vi "SensorInit.vi"(8 "error in (no error)":errorcluster, 9 "TC channel":tag="cDAQ1Mod3/ai0,cDAQ1Mod3/ai1,cDAQ1Mod3/ai2,cDAQ1Mod3/ai3,cDAQ1Mod3/ai4,cDAQ1Mod3/ai5,cDAQ1Mod3/ai6,cDAQ1Mod3/ai7", 10 "physical channels in":tag="cDAQ1Mod1/ai1,cDAQ1Mod1/ai2", 11 "Sample Rate":dbl) -> (0 "error out":errorcluster, 3 "Task out":refnum<k21>)   [LabVIEW 2020]
uses:
  <vilib>/DAQmx/create/channels.llb/DAQmx Create Channel (AI-Temperature-Thermocouple).vi
  <vilib>/DAQmx/create/channels.llb/DAQmx Create Channel (AI-Voltage-Basic).vi
  <vilib>/DAQmx/configure/timing.llb/DAQmx Timing (Sample Clock).vi
  <resource>/objmgr/daqmx.rc
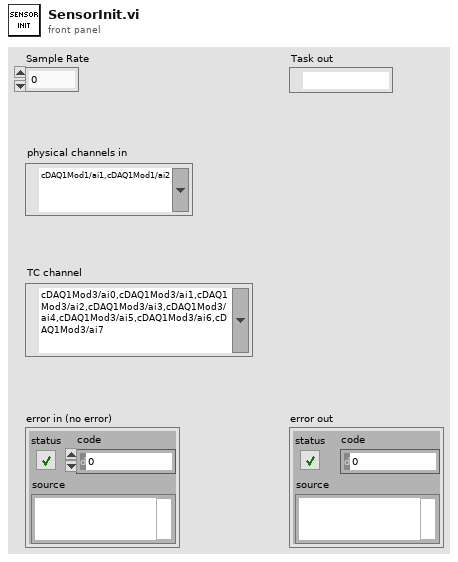
[diagram p1: front panel]
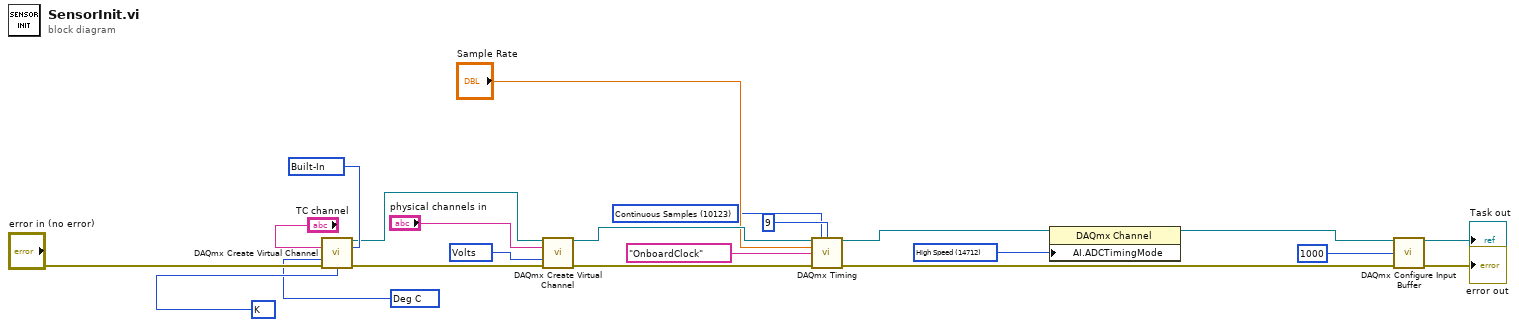
[diagram p0: block diagram]
diagram:
  w17 = 10348 items=["Volts"=10348, "From Custom Scale"=10065] ("units")
  w14 = 14712 items=["Automatic"=16097, "High Resolution"=10195, "High Speed"=14712, "Best 50 Hz Rejection"=14713, "Best 60 Hz Rejection"=14714, "Custom"=10137] ("AI.ADCTimingMode")
  w4 = 10123 items=["Finite Samples"=10178, "Continuous Samples"=10123, "Hardware Timed Single Point"=12522] ("sample mode")
  w3 = 10073 items=["J"=10072, "K"=10073, "N"=10077, "R"=10082, "S"=10085, "T"=10086, "B"=10047, "E"=10055] ("thermocouple type")
  w22 = 10200 items=["Built-In"=10200, "Constant Value"=10116, "Channel"=10113] ("cjc source")
  w2 = 10143 items=["Deg C"=10143, "Deg F"=10144, "Kelvins"=10325, "Deg R"=10145, "From Custom Scale"=10065] ("units")
  n1 = call-poly <vilib>:"DAQmx Create Virtual Channel.vi"("physical channels"="TC channel", "cjc source"=w22, "units"=w2, "error in"="error in (no error)", "thermocouple type"=w3) -> ("task out"=w18:refnum<k21>, "error out"=w19:errorcluster)  [unwired: 9 in]
  n2 = call-poly <vilib>:"DAQmx Create Virtual Channel.vi"("task in"=w18, "physical channels"="physical channels in", "units"=w17, "error in"=w19) -> ("task out"=w21:refnum<k21>, "error out"=w20:errorcluster)  [unwired: 10 in]
  n3 = call-poly <vilib>:"DAQmx Timing.vi"("task/channels in"=w21, "sample mode"=w4, "samples per channel"=9, "rate"="Sample Rate", "source"=tag "OnboardClock", "error in"=w20) -> ("task out"=w12:refnum<k21>, "error out"=w5:errorcluster)  [unwired: 8 in]
  n4 = property class="DAQmx Channel"(reference=w12, "AI.ADCTimingMode"=w14) -> (reference out=w13:refnum<k21>)  [unwired: 1 in, 1 out]
  n5 = call <vilib>:"DAQmx Configure Input Buffer.vi"("task/channels in"=w13, "buffer size (in samples per channel)"=u32 1000, "error in"=w5) -> ("task out"=→"Task out":refnum<k21>, "error out"=→"error out":errorcluster)  [unwired: 11 in]
